vi "Loop Rate.vi"() -> (3 "Loop Rate (Hz)":u32)   [LabVIEW 2010]
uses:
  <vilib>/ptbypt/NI_PtbyPt.lvlib
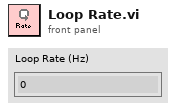
[diagram p1: front panel]
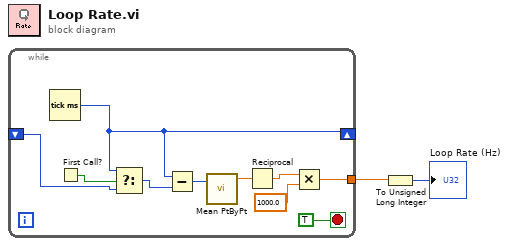
[diagram p0: block diagram]
diagram:
  n1 = while {
    shift-right: [w9] -> _
    shift-left: _ -> [w11]
    tunnel: [w4] -> w2
    stop <- TRUE stop-if-true
    n2 = Tick Count (ms)() -> (millisecond timer value=w9:u32)
    n3 = First Call?() -> (First Call?: T/F=w12:bool)
    n4 = Select(t=w9, s=w12, f=w11) -> (s? t:f=w10:u32)
    n5 = Subtract(x=w9, y=w10) -> (x-y=w8:u32)
    n6 = call <vilib>:"Mean PtByPt.vi"("x"=w8) -> ("mean"=w7:dbl)  [unwired: 3 in, 1 out]
    n7 = Reciprocal(x=w7) -> (1/x=w6:dbl)
    n8 = Multiply(x=w6, y=1000.0) -> (x*y=w4:dbl)
  }
  n9 = To Unsigned Long Integer(number=w2) -> (unsigned 32bit integer=→"Loop Rate (Hz)":u32)
